vi "Monitor ConstantSet (Core).vi"(7 "Setpoint (TEMP)":T6, 8 "error in (no error)":errorcluster, 10 "Address (0)":i32, 11 "VISA resource name":refnum<visa-resource-name>) -> (0 "error out":errorcluster, 1 "REFrigerator":T3, 2 "TEMP/HUMI":T5, 3 "VISA resource name out":refnum<visa-resource-name>, 4 "PTC":T1, 5 "RELAY":T2)   [LabVIEW 2016, in "Environment Chamber.lvlib" / "Climatic Chamber.lvlib"]
doc: "<b>Constant monitor\n(P-200, P-300 controllers only)</B>\n\nReturns the temperature, humidity, refrigerator, time signal or specimen temperature control set point in constant setup (No.1)."
uses:
  Climatic Chamber.lvlib
  Private/Type Defs/Refrigerator Mode Enum.ctl
  Private/Type Defs/Ref ConstSetting Cluster.ctl
  Private/Type Defs/Constant OptionParameter Enum.ctl
  Private/Type Defs/Temp_Humi ConstSetting Cluster.ctl
  Private/Type Defs/TimeSig ConstSetting Cluster.ctl
  Private/Type Defs/PTC ConstSetting Cluster.ctl
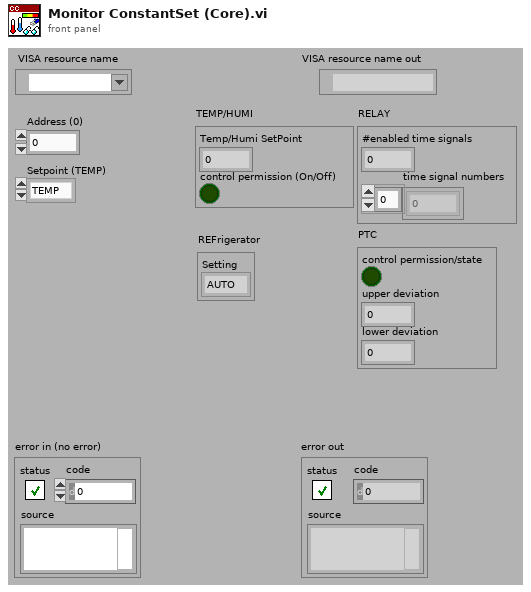
[diagram p1: front panel]
types:
  T1 = typedef "Environment Chamber.lvlib/Climatic Chamber.lvlib/PTC ConstSetting Cluster.ctl" = cluster{"control permission/state":bool, "upper deviation":dbl, "lower deviation":dbl}
  T2 = typedef "Environment Chamber.lvlib/Climatic Chamber.lvlib/TimeSig ConstSetting Cluster.ctl" = cluster{"#enabled time signals":i32, "time signal numbers":i32[]}
  T3 = typedef "Environment Chamber.lvlib/Climatic Chamber.lvlib/Ref ConstSetting Cluster.ctl" = cluster{"Setting":T4}
  T4 = typedef "Environment Chamber.lvlib/Climatic Chamber.lvlib/Refrigerator Mode Enum.ctl" = enum16{"AUTO", "OFF", "20", "50", "100"}
  T5 = typedef "Environment Chamber.lvlib/Climatic Chamber.lvlib/Temp_Humi ConstSetting Cluster.ctl" = cluster{"Temp/Humi SetPoint":dbl, "control permission (On/Off)":bool}
  T6 = typedef "Environment Chamber.lvlib/Climatic Chamber.lvlib/Constant OptionParameter Enum.ctl" = enum16{"TEMP", "HUMI", "REF", "RELAY", "PTC"}
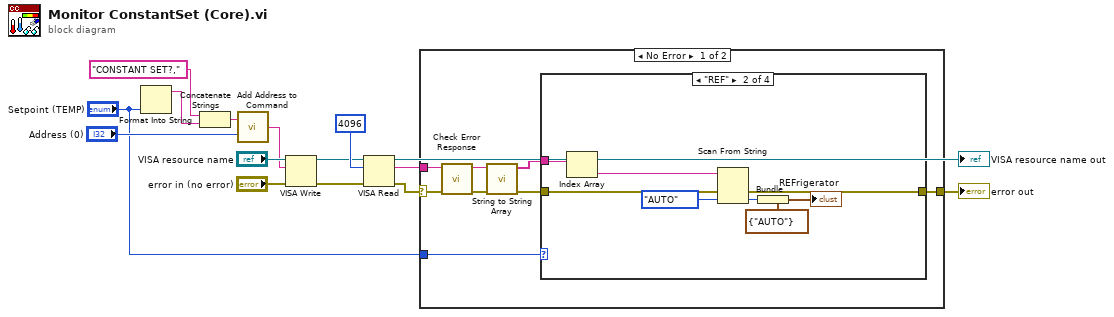
[diagram p0: block diagram]
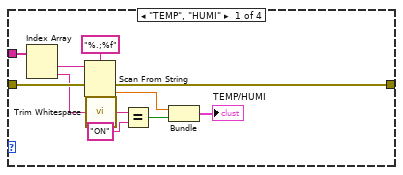
[diagram p2: hidden frame]
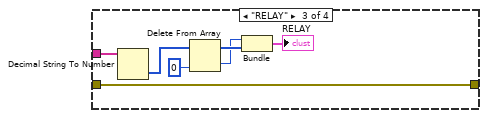
[diagram p3: hidden frame]
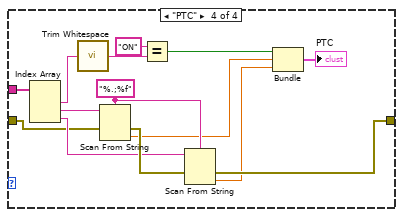
[diagram p4: hidden frame]
diagram:
  n1 = Format Into String("Setpoint (TEMP)") -> (resulting string=w2:string)  [unwired: 3 in, 1 out]
  n2 = Concatenate Strings("CONSTANT SET?,", w2) -> (w3:string)
  n3 = call "Add Address to Command.vi"("Address (0)"="Address (0)", "Command"=w3) -> ("Command OUT"=w8:string)
  n4 = VISA Write(VISA resource name="VISA resource name", write buffer=w8, error in (no error)="error in (no error)") -> (VISA resource name out=w12:refnum<visa-resource-name>, error out=w11:errorcluster)  [unwired: 1 out]
  n5 = VISA Read(VISA resource name=w12, byte count=u32 4096, error in (no error)=w11) -> (VISA resource name out=→"VISA resource name out":refnum<visa-resource-name>, read buffer=w6:string, error out=w7:errorcluster)  [unwired: 1 out]
  n6 = case shown="No Error" w7 {
    selector: w7 -> [w21 w64]
    tunnel: w6 -> [w22 _]
    tunnel: [w17 w64] -> w5
    tunnel: "Setpoint (TEMP)" -> [w16 _]
    frame No Error {
      n7 = call "Check Error Response.vi"("error in (no error)"=w21, "read String"=w22) -> ("error out"=w20:errorcluster, "String out"=w19:string)  [unwired: 7 in, 1 out]
      n8 = call "String to String Array.vi"("error in (no error)"=w20, "String received"=w19) -> ("error out"=w23:errorcluster, "Array Data"=w18:string[])  [unwired: 8 in]
      n9 = case shown="\"REF\"" w16 {
        tunnel: w23 -> [w34 w39 w48 w55]
        tunnel: w18 -> [w33 w42 w49 w62]
        tunnel: [w27 w38 w48 w54] -> w17
        frame "TEMP", "HUMI" {
          n10 = Index Array(array=w33) -> (element #1=w32:string, element #2=w30:string)  [unwired: 2 in]
          n11 = Scan From String(format string="%.;%f", input string=w32, error in=w34) -> (error out=w27:errorcluster, output 1=w25:dbl)  [unwired: 2 in, 2 out]
          n12 = call <vilib>:"Trim Whitespace.vi"("string"=w30) -> ("trimmed string"=w28:string)  [unwired: 1 in]
          n13 = Equal?(x=w28, y="ON") -> (x = y?=w26:bool)
          n14 = Bundle(w25, w26) -> (→"TEMP/HUMI":cluster{dbl, bool})  [unwired: 1 in]
        }
        frame "REF" {
          n15 = Index Array(array=w42) -> (element=w40:string)  [unwired: 1 in]
          n16 = Scan From String(input string=w40, error in=w39, default 1=Refrigerator_Mode_Enum."AUTO" ("Mode")) -> (error out=w38:errorcluster, output 1=w37:T4)  [unwired: 2 in, 2 out]
          n17 = Bundle(cluster=T3 {"Setting"=enum."AUTO"} ("REFrigerator"), "Setting"=w37) -> (→"REFrigerator":T3)
        }
        frame "RELAY" {
          n18 = Decimal String To Number(string=w49) -> (number=w47:i32[])  [unwired: 2 in, 1 out]
          n19 = Delete From Array(array=w47, index=0) -> (deleted portion=w44:i32, array with subset deleted=w45:i32[])  [unwired: 1 in]
          n20 = Bundle(w44, w45) -> (→"RELAY":cluster{i32, i32[]})  [unwired: 1 in]
        }
        frame "PTC" {
          w56 = "%.;%f" ("format string")
          n21 = Index Array(array=w62) -> (element #1=w61:string, element #2=w58:string, element #3=w57:string)  [unwired: 3 in]
          n22 = call <vilib>:"Trim Whitespace.vi"("string"=w61) -> ("trimmed string"=w60:string)  [unwired: 1 in]
          n23 = Scan From String(format string=w56, input string=w58, error in=w55) -> (error out=w63:errorcluster, output 1=w52:dbl)  [unwired: 2 in, 2 out]
          n24 = Equal?(x="ON", y=w60) -> (x = y?=w53:bool)
          n25 = Scan From String(format string=w56, input string=w57, error in=w63) -> (error out=w54:errorcluster, output 1=w51:dbl)  [unwired: 2 in, 2 out]
          n26 = Bundle(w53, w52, w51) -> (→"PTC":cluster{bool, dbl, dbl})  [unwired: 1 in]
        }
      }
    }
    frame Error {
    }
  }
  "error out" <- w5
